vi "Generate license file.vi"() -> ()   [LabVIEW 2016]
panel:
  out "error out":errorcluster
  in  "Prefix text":string="abcde"
  out "Content of the license file":string
  out "Path of the license file":path
  # "Run this VI to gereate the license file. The content is based on the information of local MAC address and the prefix text and converting into MD5 hash."
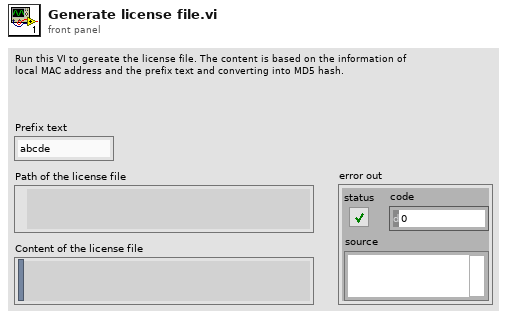
[diagram p1: front panel]
types:
  T1 = enum16{"open", "replace", "create", "open or create", "replace or create", "replace or create with confirmation"}
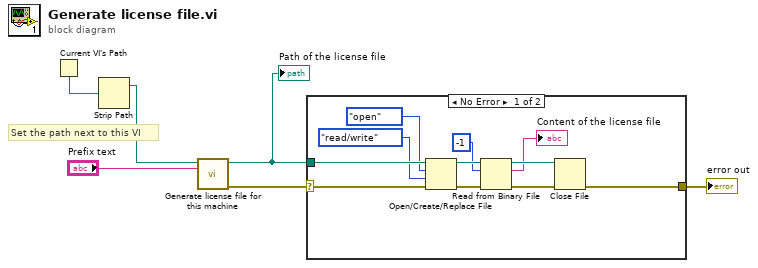
[diagram p0: block diagram]
diagram:
  # "Set the path next to this VI"
  n1 = Current VI's Path() -> (path=w5:path)
  n2 = Strip Path(path=w5) -> (stripped path=w4:path)  [unwired: 1 out]
  n3 = call "Generate license file for this machine.vi"("prefix text"="Prefix text", "folder path"=w4) -> ("error out"=w3:errorcluster, "file path"=w2:path)  [unwired: 8 in]
  "Path of the license file" <- w2
  n4 = case shown="No Error" w3 {
    selector: w3 -> [w14 w18]
    tunnel: w2 -> [w17 _]
    tunnel: [w7 w18] -> w1
    frame No Error {
      n5 = Open/Create/Replace File(file path (use dialog)=w17, error in=w14, operation (0:open)=T1."open", access (0:read/write)=enum16{"read/write", "read-only", "write-only"}."read/write") -> (refnum out=w13:refnum<file>, error out=w12:errorcluster)  [unwired: 2 in, 1 out]
      n6 = Read from Binary File(8:w12, 10:-1 ("count (1)"), 11:w13) -> (0:w11:errorcluster, 2:→"Content of the license file":string, 3:w10:refnum<file>)  [unwired: 3 in, 1 out]
      n7 = Close File(refnum=w10, error in=w11) -> (error out=w7:errorcluster)  [unwired: 1 out]
    }
    frame Error {
    }
  }
  "error out" <- w1
